vi "List Objects.vi"(7 "Max keys":u32, 8 "error in (no error)":errorcluster, 9 "Delimiter":string, 10 "Prefix":string, 11 "Bucket in":refnum<class "Bucket.lvclass">) -> (0 "error out":errorcluster, 1 "Common Prefixes":string[](array[string]), 2 "Objects":T1[](array[typedef]), 3 "Bucket out":refnum<class "Bucket.lvclass">)   [LabVIEW 2015, in "NI_AWS_S3.lvlib" / "Bucket.lvclass"]
doc: "This implementation of the GET operation returns some or all (up to 1,000) of the objects in a bucket."
uses:
  Bucket.lvclass
  Object Content.ctl
  Storage Class.ctl
  Owner.ctl
  NI_AWS_S3.lvlib
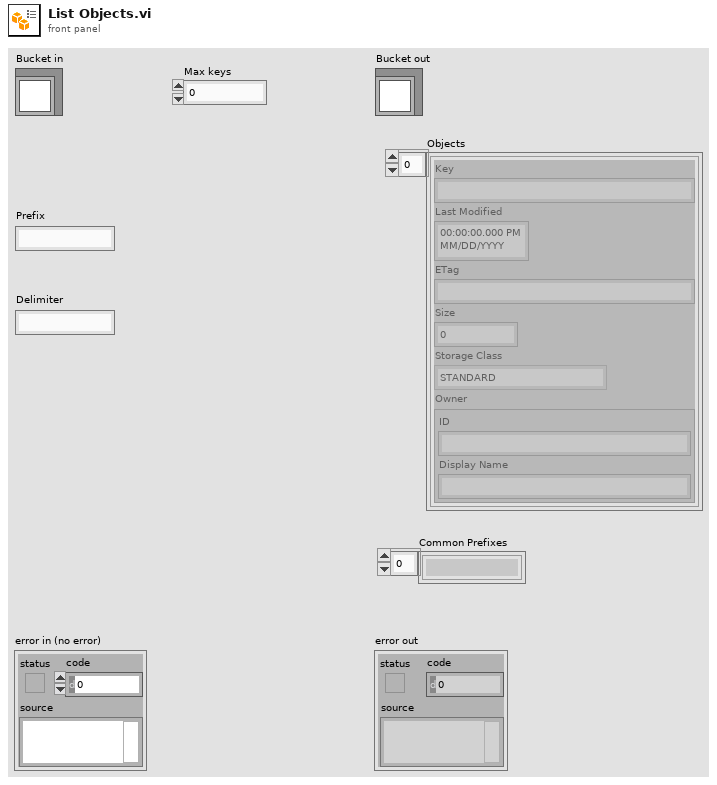
[diagram p1: front panel]
types:
  T1 = typedef "NI_AWS_S3.lvlib/Object Content.ctl" = cluster{"Key":string, "Last Modified":timestamp, "ETag":string, "Size":u64, "Storage Class":T2, "Owner":T3}
  T2 = typedef "NI_AWS_S3.lvlib/Storage Class.ctl" = enum16{"STANDARD", "REDUCED_REDUNDANCY"}
  T3 = typedef "NI_AWS_S3.lvlib/Owner.ctl" = cluster{"ID":string, "Display Name":string}
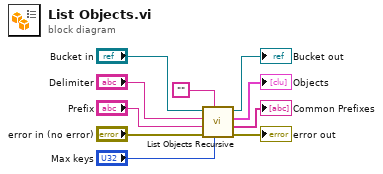
[diagram p0: block diagram]
diagram:
  n1 = call "List Objects Recursive.vi"("Remaining objs"="Max keys", "marker"="", "error in (no error)"="error in (no error)", "Prefix"="Prefix", "Delimiter"="Delimiter", "Bucket in"="Bucket in") -> ("error out"=→"error out":errorcluster, "Common Prefixes"=→"Common Prefixes":string[], "Objects"=→"Objects":T1[], "Bucket out"=→"Bucket out":refnum<class "Bucket.lvclass">)  [unwired: 2 in]
